vi "Dequeue Message.vi"(8 "error in (no error)":errorcluster[](array[cluster]), 11 "Message Queue":refnum<queue>) -> (0 "error out":errorcluster[](array[cluster]), 1 "Message Data":variant, 2 "Message":string, 3 "dup Message Queue":refnum<queue>)   [LabVIEW 2018, in "Message Queue.lvlib"]
doc: "This VI pulls messages off the Message Queue."
uses:
  Message Queue.lvlib
  Message Cluster.ctl
  <userlib>/NIST/NISTErrorLib/NISTErrorLib.lvlib
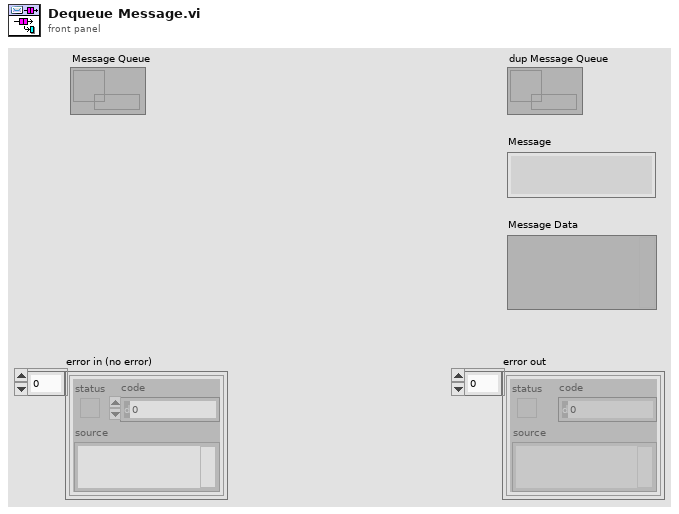
[diagram p1: front panel]
types:
  T1 = typedef "Message Queue.lvlib/Message Cluster.ctl" = cluster{"Message":string, "Message Data":variant}
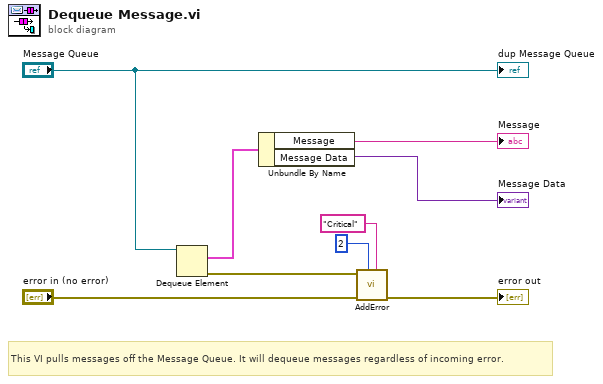
[diagram p0: block diagram]
diagram:
  # "This VI pulls messages off the Message Queue. It will dequeue messages regardless of incoming error."
  n1 = Dequeue Element(queue="Message Queue") -> (element=w6:T1, error out=w3:errorcluster)  [unwired: 2 in, 2 out]
  n2 = Unbundle By Name(w6) -> ("Message"=→"Message":string, "Message Data"=→"Message Data":variant)
  n3 = call <userlib>:"AddError.vi"("Severity"="Critical", "Priority"=u8 2, "ErrorArray In"="error in (no error)", "error in (no error)"=w3) -> ("ErrorArray Out"=→"error out":errorcluster[])  [unwired: 6 in, 1 out]
  "dup Message Queue" <- "Message Queue"
